vi "Convert Steering Frame Velocity to Arc Velocity.vi"(11 "steering frame velocity":dbl[](array[numeric])) -> (3 "arc velocity":T1={"turning radius"=1.0, "tangential velocity"=0.0, "angle from tangent (rad)"=0.0})   [LabVIEW 2017, in "NI_Robotics_Steering Frame.lvclass"]
uses:
  <vilib>/robotics/Steering/Steering Frame/NI_Robotics_Steering Frame.lvclass
  <vilib>/robotics/Steering/Steering Frame/Arc Velocity.ctl
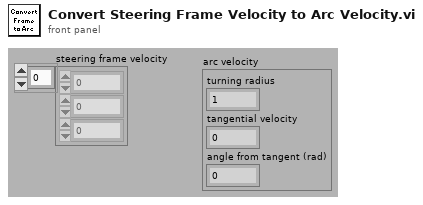
[diagram p1: front panel]
types:
  T1 = typedef "NI_Robotics_Steering Frame.lvclass/Arc Velocity.ctl" = cluster{"turning radius":dbl, "tangential velocity":dbl, "angle from tangent (rad)":dbl}
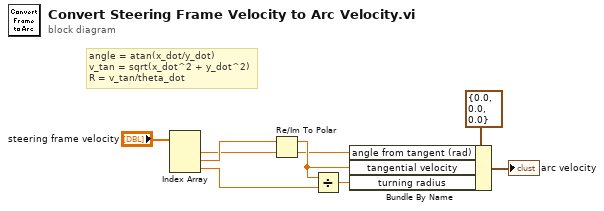
[diagram p0: block diagram]
diagram:
  # "angle = atan(x_dot/y_dot)\nv_tan = sqrt(x_dot^2 + y_dot^2)\nR = v_tan/theta_dot"
  n1 = Index Array(array="steering frame velocity") -> (element #1=w3:dbl, element #2=w4:dbl, element #3=w7:dbl)  [unwired: 3 in]
  n2 = Re/Im To Polar(2:w3, 3:w4) -> (0:w1:dbl, 1:w2:dbl)
  n3 = Divide(x=w2, y=w7) -> (x/y=w6:dbl)
  n4 = Bundle By Name(cluster=T1 {"turning radius"=0.0, "tangential velocity"=0.0, "angle from tangent (rad)"=0.0} ("arc velocity"), "angle from tangent (rad)"=w1, "tangential velocity"=w2, "turning radius"=w6) -> (→"arc velocity":T1)
